vi "error code parser.vi"(2 "device":u8, 3 "Error":errorcluster, 4 "Status":u8 format="%.0x") -> (0 "Error out":errorcluster)   [LabVIEW 2013, in "dynamic profibus.lvlib"]
uses:
  dynamic profibus.lvlib
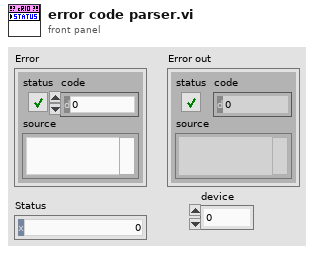
[diagram p1: front panel]
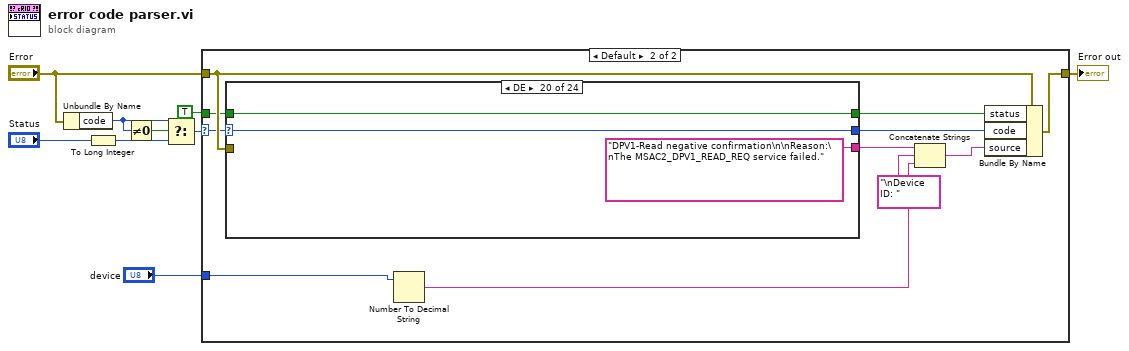
[diagram p0: block diagram]
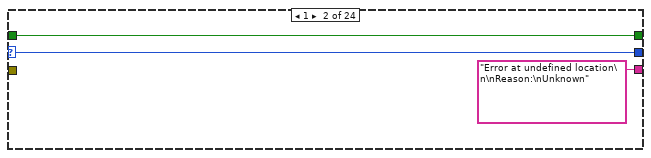
[diagram p4: hidden frame]
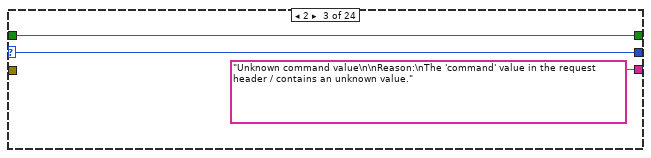
[diagram p5: hidden frame]
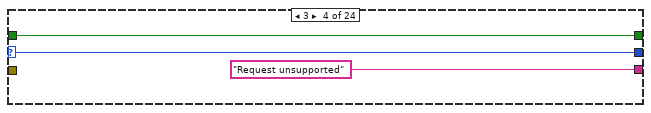
[diagram p6: hidden frame]
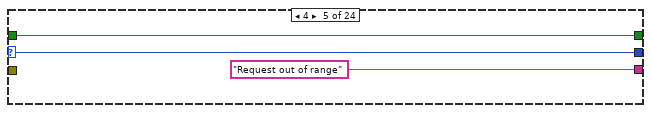
[diagram p7: hidden frame]
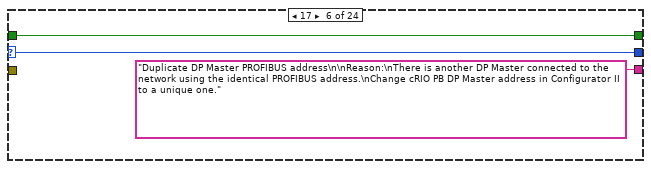
[diagram p8: hidden frame]
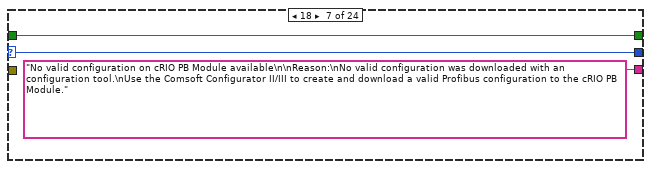
[diagram p9: hidden frame]
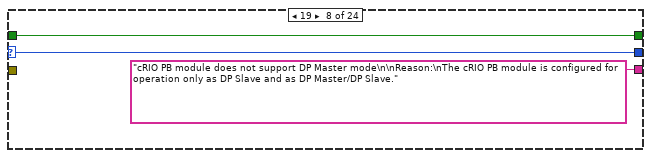
[diagram p10: hidden frame]
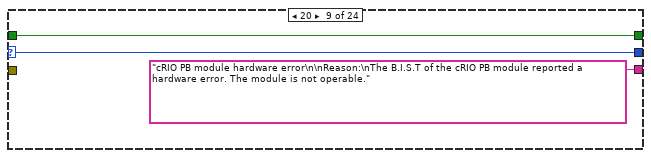
[diagram p11: hidden frame]
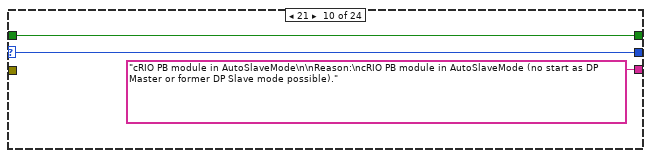
[diagram p12: hidden frame]
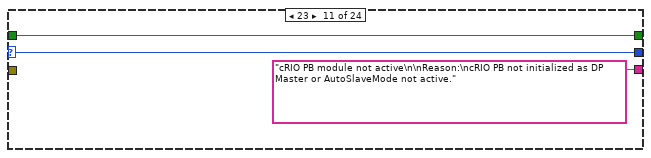
[diagram p13: hidden frame]
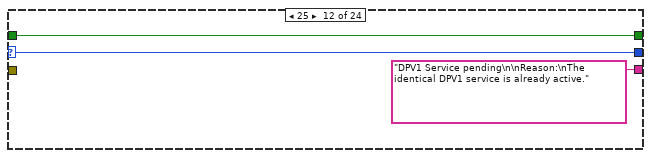
[diagram p14: hidden frame]
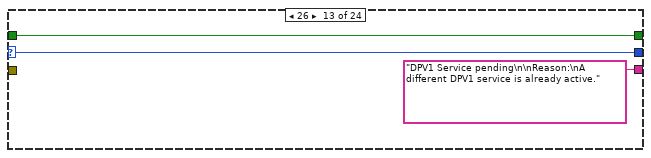
[diagram p15: hidden frame]
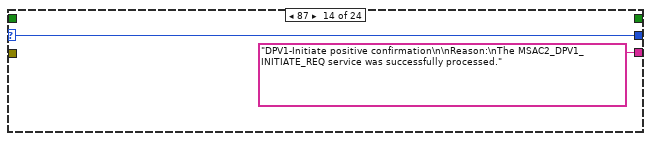
[diagram p16: hidden frame]
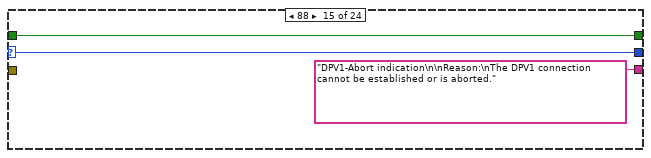
[diagram p17: hidden frame]
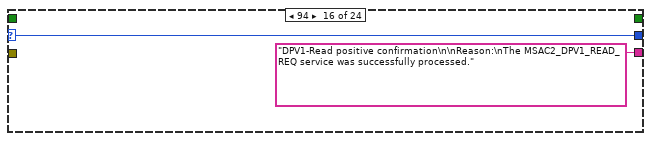
[diagram p18: hidden frame]
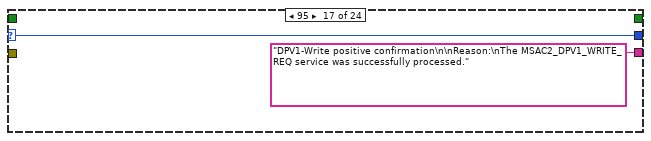
[diagram p19: hidden frame]
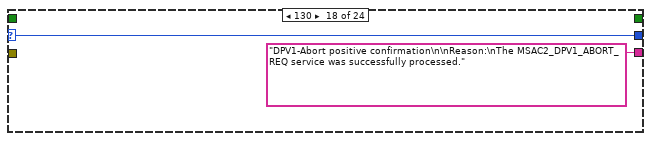
[diagram p20: hidden frame]
diagram:
  n1 = Unbundle By Name("Error") -> ("code"=w8:i32)
  n2 = To Long Integer(number="Status") -> (32bit integer=w7:i32)
  n3 = Not Equal To 0?(x=w8) -> (x != 0?=w9:bool)
  n4 = Select(t=w8, s=w9, f=w7) -> (s? t:f=w6:i32)
  n5 = case shown="Default" w6 {
    selector: w6 -> [_ w16]
    tunnel: "Error" -> [w10 w21]
    tunnel: [w10 w20] -> w5
    tunnel: TRUE -> [_ w19]
    tunnel: "device" -> [_ w13]
    frame 0 {
    }
    frame Default {
      n6 = case shown="DE" w16 {
        selector: w16 -> [_ w24 w27 w30 w33 w36 w39 w42 w45 w48 w51 w54 w57 w59 w62 w64 w66 w68 w71 w74 w77 w80 w83 w87]
        tunnel: w19 -> [_ w22 w25 w28 w31 w34 w37 w40 w43 w46 w49 w52 w55 _ w60 _ _ _ w69 w72 w75 w78 w81 w86]
        tunnel: [_ w24 w27 w30 w33 w36 w39 w42 w45 w48 w51 w54 w57 w59 w62 w64 w66 w68 w71 w74 w77 w80 w83 w87] -> w18
        tunnel: [_ "Error at undefined location\n\nReason:\nUnknown" "Unknown command value\n\nReason:\nThe 'command' value in the request header / contains an unknown value." "Request unsupported" "Request out of range" "Duplicate DP Master PROFIBUS address\n\nReason:\nThere is another DP Master connected to the network using the identical PROFIBUS address.\nChange cRIO PB DP Master address in Configurator II to a unique one." "No valid configuration on cRIO PB Module available\n\nReason:\nNo valid configuration was downloaded with an configuration tool.\nUse the Comsoft Configurator II/III to create and download a valid Profibus configuration to the cRIO PB Module." "cRIO PB module does not support DP Master mode\n\nReason:\nThe cRIO PB module is configured for operation only as DP Slave and as DP Master/DP Slave." "cRIO PB module hardware error\n\nReason:\nThe B.I.S.T of the cRIO PB module reported a hardware error. The module is not operable." "cRIO PB module in AutoSlaveMode\n\nReason:\ncRIO PB module in AutoSlaveMode (no start as DP Master or former DP Slave mode possible)." "cRIO PB module not active\n\nReason:\ncRIO PB not initialized as DP Master or AutoSlaveMode not active." "DPV1 Service pending\n\nReason:\nThe identical DPV1 service is already active." "DPV1 Service pending\n\nReason:\nA different DPV1 service is already active." "DPV1-Initiate positive confirmation\n\nReason:\nThe MSAC2_DPV1_INITIATE_REQ service was successfully processed." "DPV1-Abort indication\n\nReason:\nThe DPV1 connection cannot be established or is aborted." "DPV1-Read positive confirmation\n\nReason:\nThe MSAC2_DPV1_READ_REQ service was successfully processed." "DPV1-Write positive confirmation\n\nReason:\nThe MSAC2_DPV1_WRITE_REQ service was successfully processed." "DPV1-Abort positive confirmation\n\nReason:\nThe MSAC2_DPV1_ABORT_REQ service was successfully processed." "DPV1-Initiate negative confirmation\n\nReason:\nThe DPV1 connection cannot be established." "DPV1-Read negative confirmation\n\nReason:\nThe MSAC2_DPV1_READ_REQ service failed." "DPV1-Write negative confirmation\n\nReason:\nThe MSAC2_DPV1_WRITE_REQ service failed." "DP Slave is not in state DataExchange, the output data are not processed, the input data are not valid\n\nReason:\nDP Slave is wrongly configured or DP Slave does not respond." "DP Slave is in state DataExchange but reports external diagnostic data\n\nReason:\nDP Slave detected manufacturer specific error i.e. a broken wire on an input channel.\nReceive and analyze DP Slave related diagnostic information." w84] -> w15
        tunnel: [_ w22 w25 w28 w31 w34 w37 w40 w43 w46 w49 w52 w55 _ w60 _ _ _ w69 w72 w75 w78 w81 w86] -> w17
        tunnel: w21 -> [_ _ _ _ _ _ _ _ _ _ _ _ _ _ _ _ _ _ _ _ _ _ _ w85]
        frame 0 {
        }
        frame 1 {
        }
        frame 2 {
        }
        frame 3 {
        }
        frame 4 {
        }
        frame 17 {
        }
        frame 18 {
        }
        frame 19 {
        }
        frame 20 {
        }
        frame 21 {
        }
        frame 23 {
        }
        frame 25 {
        }
        frame 26 {
        }
        frame 87 {
        }
        frame 88 {
        }
        frame 94 {
        }
        frame 95 {
        }
        frame 130 {
        }
        frame 215 {
        }
        frame 222 {
        }
        frame 223 {
        }
        frame 195 {
        }
        frame 255 {
        }
        frame Default {
          n7 = Unbundle By Name(w85) -> ("source"=w84:string)
        }
      }
      n8 = Number To Decimal String(number=w13) -> (decimal integer string=w12:string)  [unwired: 1 in]
      n9 = Concatenate Strings(w15, "\nDevice ID: " ("string"), w12) -> (w14:string)
      n10 = Bundle By Name(cluster=w21, "status"=w17, "code"=w18, "source"=w14) -> (w20:errorcluster)
    }
  }
  "Error out" <- w5
